vi "Process Increment.vi"(11 "station #":i32) -> (3 "error":bool)   [LabVIEW 2019]
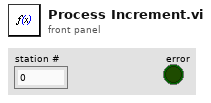
[diagram p1: front panel]
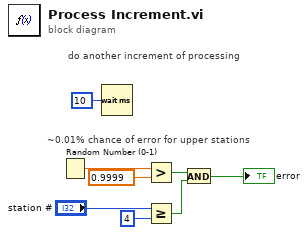
[diagram p0: block diagram]
diagram:
  # "~0.01% chance of error for upper stations"
  # "do another increment of processing"
  n1 = Random Number (0-1)() -> (number: 0 to 1=w7:dbl)
  n2 = Wait (ms)(milliseconds to wait=u32 10) -> ()  [unwired: 1 out]
  n3 = Greater?(x=w7, y=0.9999) -> (0:w6:bool)
  n4 = Greater Or Equal?(x="station #", y=4) -> (x >= y?=w1:bool)
  n5 = And(x=w6, y=w1) -> (x .and. y?=→"error":bool)
